vi "click_event.vi"(5 "start2 2":refnum<vi>, 7 "start1 2":refnum<vi>, 9 "focus row":dbl, 10 "checkbox array in":i32[](array[numeric]), 11 "MulticolumnListbox in":refnum<vi>) -> (0 "Boolean":bool, 2 "FocusRow":i32, 3 "checkbox array out":i32[](array[numeric]))   [LabVIEW 2015]
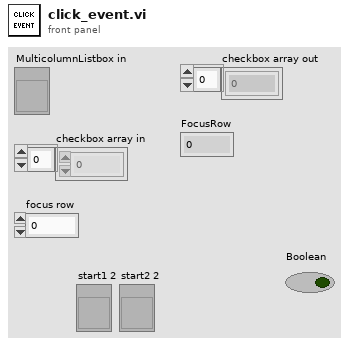
[diagram p1: front panel]
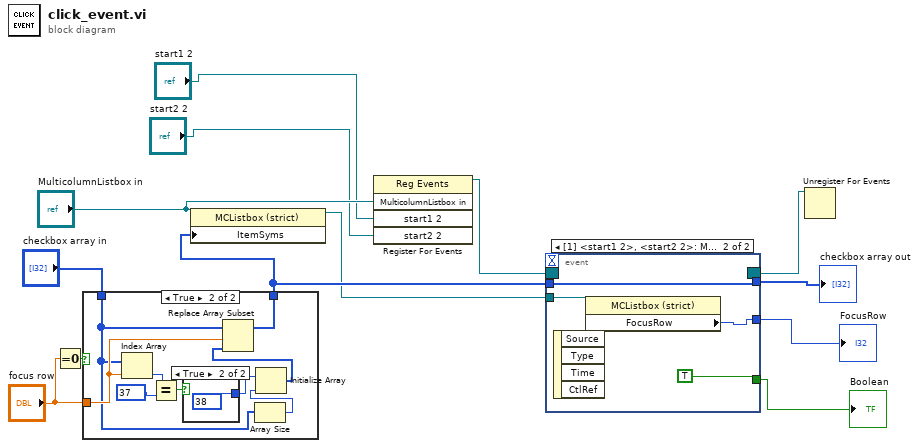
[diagram p0: block diagram]
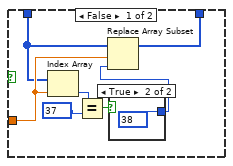
[diagram p2: hidden frame]
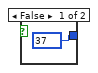
[diagram p3: hidden frame]
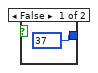
[diagram p4: hidden frame]
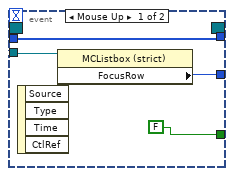
[diagram p5: hidden frame]
diagram:
  n1 = Equal To 0?(x="focus row") -> (x = 0?=w2:bool)
  n2 = case shown="True" w2 {
    tunnel: "focus row" -> [w19 w31]
    tunnel: "checkbox array in" -> [w18 w25]
    tunnel: [w17 w30] -> w12
    frame False {
      n3 = Index Array(array=w18, index=w19) -> (element=w16:i32)
      n4 = Equal?(x=w16, y=37) -> (x = y?=w14:bool)
      n5 = case shown="True" w14 {
        tunnel: [37 38] -> w20
        frame False {
        }
        frame True {
        }
      }
      n6 = Replace Array Subset(array=w18, new element=w20, index=w19) -> (w17:i32[])
    }
    frame True {
      n7 = Index Array(array=w25, index=w31) -> (element=w29:i32)
      n8 = Equal?(x=w29, y=37) -> (x = y?=w27:bool)
      n9 = case shown="True" w27 {
        tunnel: [37 38] -> w26
        frame False {
        }
        frame True {
        }
      }
      n10 = Array Size(array=w25) -> (size(s)=w24:i32)
      n11 = Initialize Array(w26, w24) -> (w23:i32[])
      n12 = Replace Array Subset(array=w25, new element=w23, index=w31) -> (w30:i32[])
    }
  }
  n13 = property on="Property Node" class="MCListbox (strict)"(reference="MulticolumnListbox in", "ItemSyms"=w12) -> (reference out=w9:refnum<vi>)  [unwired: 1 in, 1 out]
  n14 = register-events("MulticolumnListbox in", "start1 2", "start2 2") -> (reference out=w7:refnum<event-registration>)  [unwired: 2 in, 1 out]
  n15 = event shown="[1] <start1 2>, <start2 2>: Mouse Up" {
    selector: w7 -> [_ _]
    dyn-events: [_ _] -> w6
    timeout: _ -> [_ _]
    tunnel: [w37 w40] -> w10
    tunnel: [w36 w38] -> w11
    tunnel: w12 -> [w37 w40]
    tunnel: w9 -> [w35 w39]
    tunnel: [FALSE TRUE] -> w3
    event Mouse Up {
      n16 = event-data() -> ()  [unwired: 1 in, 4 out]
      n17 = property on="Property Node" class="MCListbox (strict)"(reference=w35) -> ("FocusRow"=w36:i32)  [unwired: 1 in, 2 out]
    }
    event Mouse Up {
      n18 = event-data() -> ()  [unwired: 1 in, 4 out]
      n19 = property on="Property Node" class="MCListbox (strict)"(reference=w39) -> ("FocusRow"=w38:i32)  [unwired: 1 in, 2 out]
    }
  }
  "FocusRow" <- w11
  "checkbox array out" <- w10
  "Boolean" <- w3
  n20 = Unregister For Events(event registration refnum=w6) -> ()  [unwired: 1 in, 1 out]
